vi "ti2_setZPos.vi"(8 "error in (no error)":errorcluster, 11 "z Position (um)":dbl) -> (0 "error out":errorcluster)   [LabVIEW 2023, in "ti2lv.lvlib"]
uses:
  ti2lv.lvlib
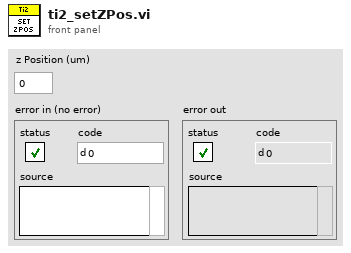
[diagram p1: front panel]
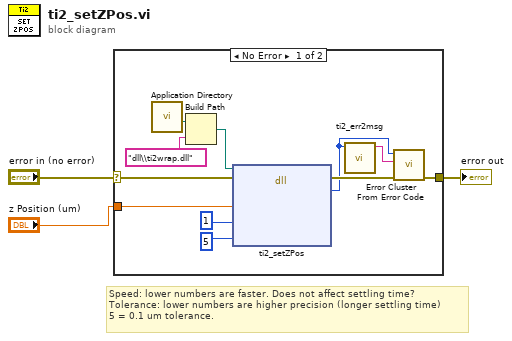
[diagram p0: block diagram]
diagram:
  # "Speed: lower numbers are faster. Does not affect settling time?\nTolerance: lower numbers are higher precision (longer settling time)\n5 = 0.1 um tolerance."
  n1 = case shown="No Error" "error in (no error)" {
    selector: "error in (no error)" -> [w13 w15]
    tunnel: [w14 w15] -> w3
    tunnel: "z Position (um)" -> [w9 _]
    frame No Error {
      n2 = call <vilib>:"Application Directory.vi"() -> ("Application Directory"=w7:path)
      n3 = Build Path(base path=w7, name or relative path="dll\\ti2wrap.dll") -> (appended path=w6:path)
      n4 = dll-call lib="?" fn="ti2_setZPos"(path in=w6, error in=w13, "zPos_um"=w9, "speed"=1 ("tolerance"), "tolerance"=5) -> (error out=w12:errorcluster, "return type"=w11:i32)  [unwired: 4 in, 1 out]
      n5 = call "ti2_err2msg.vi"("Error Code"=w11) -> ("Error Message"=w10:string)  [unwired: 10 in]
      n6 = call <vilib>:"Error Cluster From Error Code.vi"("error in (no error)"=w12, "error message (\"\")"=w10, "error code (0)"=w11) -> ("error out"=w14:errorcluster)  [unwired: 6 in]
    }
    frame Error {
    }
  }
  "error out" <- w3
